vi "gcf_n.vi"(11 "Values":i32[](array[numeric])=[0, 0, 0, 0, 0, 0, 0, 0, 0, 0]) -> (3 "GCF":i32)   [LabVIEW 2009]
doc: "Finds the GCF of numbers in an array. Disregards negatives and zeroes.\nUses the functions \"GCF(2)\", \"turn negatives to zeroes\", and \"strip zeroes\"."
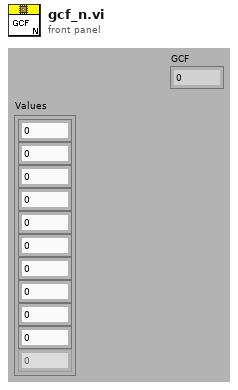
[diagram p1: front panel]
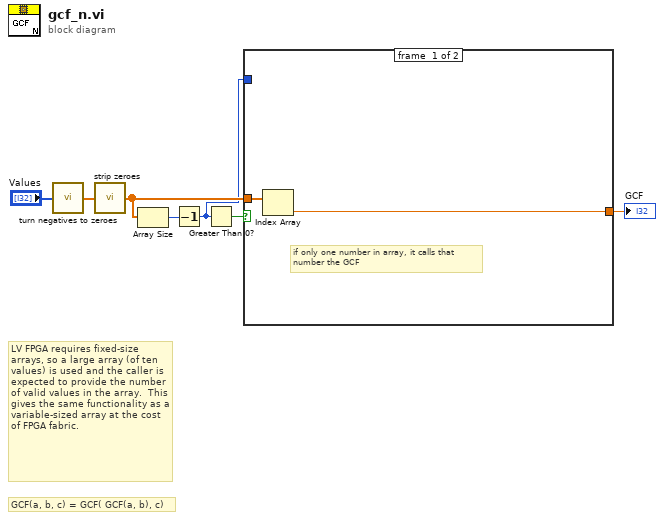
[diagram p0: block diagram]
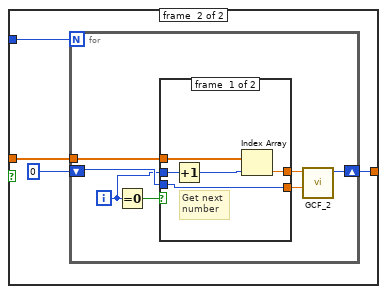
[diagram p2: hidden frame]
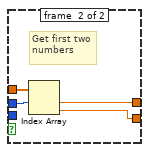
[diagram p3: hidden frame]
diagram:
  # "LV FPGA requires fixed-size arrays, so a large array (of ten values) is used and the caller is expected to provide the number of valid values in the array.  This gives the same functionality as a variable-sized array at the cost of FPGA fabric."
  # "GCF(a, b, c) = GCF( GCF(a, b), c)"
  n1 = call "turn negatives to zeroes.vi"("Array in"="Values") -> ("Array out"=w5:dbl[])
  n2 = call "strip zeroes.vi"("Array in"=w5) -> ("Array out"=w7:dbl[])
  n3 = Array Size(array=w7) -> (size(s)=w3:i32)
  n4 = Decrement(x=w3) -> (x-1=w2:i32)
  n5 = Greater Than 0?(x=w2) -> (x > 0?=w1:bool)
  n6 = case shown="False" w1 {
    tunnel: w7 -> [w9 w12]
    tunnel: [w8 w11] -> w4
    tunnel: w2 -> [_ w10]
    frame #0 {
      # "if only one number in array, it calls that\nnumber the GCF"
      n7 = Index Array(array=w9) -> (element=w8:dbl)  [unwired: 1 in]
    }
    frame #1 {
      n8 = for {
        N: w10 -> [_]
        tunnel: w12 -> [w20]
        shift-right: [w15] -> w11
        shift-left: 0 ("GCF") -> [w18]
        i -> [w16]
        n9 = Equal To 0?(x=w16) -> (x = 0?=w17:bool)
        n10 = case shown="False" w17 {
          tunnel: w20 -> [w25 w29]
          tunnel: [w22 w28] -> w14
          tunnel: [w23 w26] -> w19
          tunnel: w18 -> [w23 _]
          tunnel: w16 -> [w24 w27]
          frame #0 {
            # "Get next number"
            n11 = Increment(x=w24) -> (x+1=w21:i32)
            n12 = Index Array(array=w25, index=w21) -> (element=w22:dbl)
          }
          frame #1 {
            # "Get first two numbers"
            n13 = Index Array(array=w29, index #1=w27) -> (element #1=w28:dbl, element #2=w26:dbl)  [unwired: 1 in]
          }
        }
        n14 = call "GCF_2.vi"("B"=w19, "A"=w14) -> ("GCF"=w15:i32)  [unwired: 9 out]
      }
    }
  }
  "GCF" <- w4
